vi "workbook.create_commit.vi"(8 "error in":errorcluster, 11 "WorkbookCreateStaging in":refnum<class "WorkbookCreateStaging.lvclass">) -> (0 "error out":errorcluster, 3 "WorkbookCreateStaging out":refnum<class "WorkbookCreateStaging.lvclass">)   [LabVIEW 2020, in "WorkbookCreateStaging.lvclass"]
doc: "Creates the staged workbook from the given template and returns a handle to it."
uses:
  WorkbookCreateStaging.lvclass
  WorkbookCreateStaging.lvclass/WorkbookCreateStaging.ctl
  client.lvlib
panel:
  out "out_workbook out":i32
  in  "template_":i32
  in  "staging":i32
  in  "out_workbook":i32
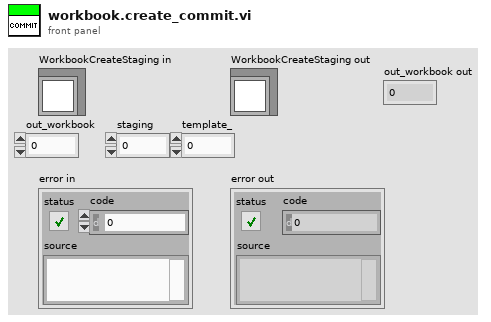
[diagram p1: front panel]
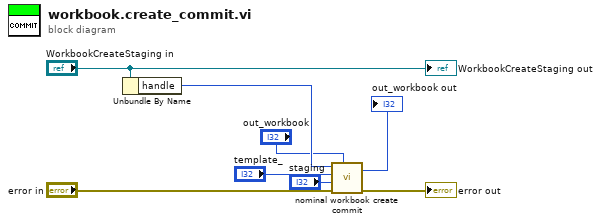
[diagram p0: block diagram]
diagram:
  n1 = Unbundle By Name("WorkbookCreateStaging in") -> ("handle"=w6:i32)
  n2 = call "nominal workbook create commit.vi"("out_workbook"="out_workbook", "error in (no error)"="error in", "staging"="staging", "template_"="template_", "client"=w6) -> ("error out"=→"error out":errorcluster, "out_workbook out"=→"out_workbook out":i32)  [unwired: 4 in, 1 out]
  "WorkbookCreateStaging out" <- "WorkbookCreateStaging in"
